vi "vipmGetInstalled.vi"   [LabVIEW 2014, in "vipm-build-tools.lvlib"]
uses:
  vipm-build-tools.lvlib
  <vilib>/JKI/VIPM API/VIPM API_vipm_api.lvlib
  <vilib>/Wiresmith Technology/LabVIEW CLI/CLI Class/CLI.lvclass
types:
  T1 = enum16{"open", "replace", "create", "open or create", "replace or create", "replace or create with confirmation"}
  T2 = typedef "VIPM API_vipm_api.lvlib/Library Contents Cluster_vipm_api.ctl" = cluster{"Package Name":string, "Version":string, "Display Name":string, "Repository Name":string, "Company Name":string, "License Type":string, "Installed":bool, "Deprecated":bool, "Dependency or Conflict Problem":bool, "Downloaded":bool}
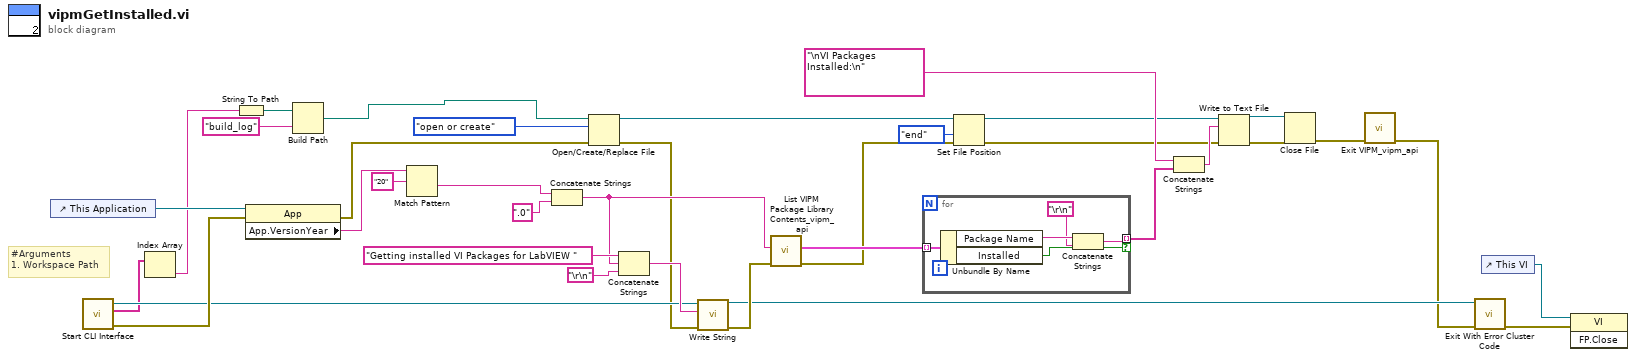
[diagram p0: block diagram]
diagram:
  # "#Arguments\n1. Workspace Path"
  n1 = control-ref of="This Application"() -> (w36:refnum<vi>)
  n2 = call <vilib>:"Start CLI Interface.vi"() -> ("error out"=w31:errorcluster, "Custom Parameters"=w24:string[], "CLI out"=w25:refnum<class "CLI.lvclass">)  [unwired: 9 in]
  n3 = Index Array(array=w24) -> (element=w23:string)  [unwired: 1 in]
  n4 = String To Path(string=w23) -> (path=w10:path)
  n5 = property class="App"(reference=w36, error in=w31) -> (error out=w21:errorcluster, "App.VersionYear"=w35:string)  [unwired: 1 out]
  n6 = Build Path(base path=w10, name or relative path="build_log") -> (appended path=w9:path)
  n7 = Match Pattern(string=w35, regular expression="20") -> (after substring=w32:string)  [unwired: 1 in, 3 out]
  n8 = Concatenate Strings(w32, ".0" ("format string")) -> (w26:string)
  n9 = Open/Create/Replace File(file path (use dialog)=w9, error in=w21, operation (0:open)=T1."open or create") -> (refnum out=w4:refnum<file>, error out=w11:errorcluster)  [unwired: 3 in, 1 out]
  n10 = Concatenate Strings("Getting installed VI Packages for LabVIEW " ("Text to Write"), w26, "\r\n") -> (w30:string)
  n11 = call <vilib>:"Write String.vi"("error in (no error)"=w11, "Text to Write"=w30, "CLI in"=w25) -> ("error out"=w27:errorcluster, "CLI out"=w18:refnum<class "CLI.lvclass">)  [unwired: 7 in]
  n12 = call <vilib>:"List VIPM Package Library Contents_vipm_api.vi"("error in (no error)"=w27, "LabVIEW Version"=w26) -> ("error out"=w5:errorcluster, "Library Contents []"=w19:T2[])  [unwired: 8 in]
  n13 = for {
    tunnel: w19 -> [w41] mode=indexing
    tunnel: [w37] -> w15 mode=indexing if=w40
    n14 = Unbundle By Name(w41) -> ("Package Name"=w39:string, "Installed"=w40:bool)
    n15 = Concatenate Strings(w39, "\r\n") -> (w37:string)
  }
  n16 = Set File Position(refnum=w4, from (0:start)=enum16{"start", "end", "current"}."end", error in=w5) -> (refnum out=w2:refnum<file>, error out=w1:errorcluster)  [unwired: 1 in]
  n17 = Concatenate Strings("\nVI Packages Installed:\n" ("string"), w15) -> (w7:string)
  n18 = Write to Text File(file (use dialog)=w2, text=w7, error in=w1) -> (refnum out=w8:refnum<file>, error out=w6:errorcluster)  [unwired: 1 in, 1 out]
  n19 = Close File(refnum=w8, error in=w6) -> (error out=w13:errorcluster)  [unwired: 1 out]
  n20 = call <vilib>:"Exit VIPM_vipm_api.vi"("error in (no error)"=w13) -> ("error out"=w12:errorcluster)  [unwired: 10 in]
  n21 = call <vilib>:"Exit With Error Cluster Code.vi"("error in (no error)"=w12, "CLI in"=w18) -> ("error out"=w17:errorcluster)  [unwired: 9 in]
  n22 = control-ref of="This VI"() -> (w16:refnum<vi>)
  n23 = invoke class="VI" method="FP.Close"(reference=w16, error in=w17) -> ()  [unwired: 1 in, 3 out]
